vi "Doc_Builder_Write_Description.vi"(10 "input item file path":path, 11 "NI_report in":refnum<class "NI_report.lvclass">) -> (3 "NI_report out":refnum<class "NI_report.lvclass">)   [LabVIEW 2019]
uses:
  <vilib>/Utility/NIReport.llb/NI_report.lvclass
  <vilib>/printing/ReportDocExtensions.llb/Append VI Description to Report (path).vi
  <vilib>/Utility/NIReport.llb/NI_ReportGenerationCore.lvlib
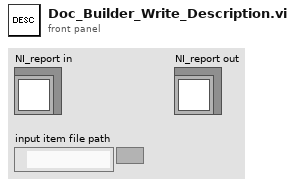
[diagram p1: front panel]
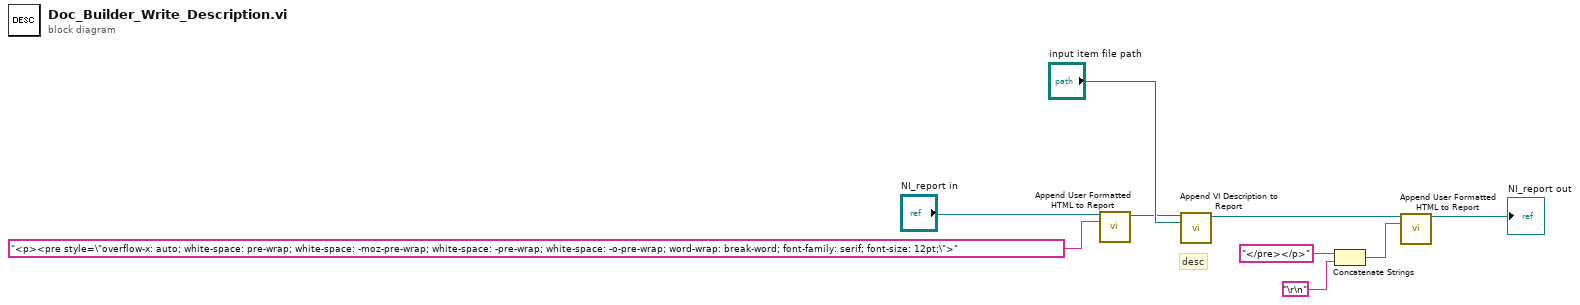
[diagram p0: block diagram]
diagram:
  # "desc"
  n1 = call-dynamic "Append User Formatted HTML to Report.vi"("report in"="NI_report in", "HTML text"="<p><pre style=\"overflow-x: auto; white-space: pre-wrap; white-space: -moz-pre-wrap; white-space: -pre-wrap; white-space: -o-pre-wrap; word-wrap: break-word; font-family: serif; font-size: 12pt;\">" ("text")) -> ("report out"=w2:refnum<class "NI_report.lvclass">)  [unwired: 12 in, 1 out]
  n2 = call-poly <vilib>:"Append VI Description to Report.vi"("report in"=w2, "VI"="input item file path") -> ("report out"=w5:refnum<class "NI_report.lvclass">)  [unwired: 9 in, 4 out]
  n3 = Concatenate Strings("</pre></p>" ("text"), "\r\n") -> (w3:string)
  n4 = call-dynamic "Append User Formatted HTML to Report.vi"("report in"=w5, "HTML text"=w3) -> ("report out"=→"NI_report out":refnum<class "NI_report.lvclass">)  [unwired: 12 in, 1 out]
